vi "UTIL Generate Analog Output.vi"(6 "sampling info":cluster{"Fs":dbl, "#s":dbl}={"Fs"=1000.0, "#s"=1000.0} {"Fs" format="%.2p"}, 8 "error in (no error)":errorcluster, 9 "frequency":dbl=10.0 format="%0.2p", 10 "amplitude":dbl=1.0 format="%0.2p", 11 "task/channels in":refnum<k21>) -> (0 "error out":errorcluster, 3 "task out":refnum<k21>)   [LabVIEW 2010]
uses:
  <vilib>/DAQmx/write.llb/DAQmx Write (Analog Wfm 1Chan NSamp).vi
  <vilib>/daqmx/miscellaneous.llb/DAQmx Fill In Error Info.vi
  <vilib>/measure/NI_MABase.lvlib
panel:
  in  "stop":bool
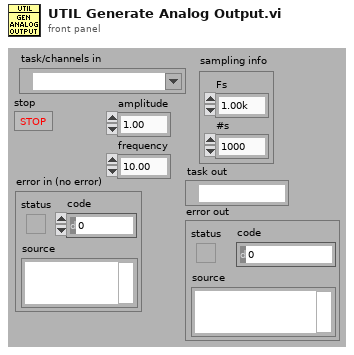
[diagram p1: front panel]
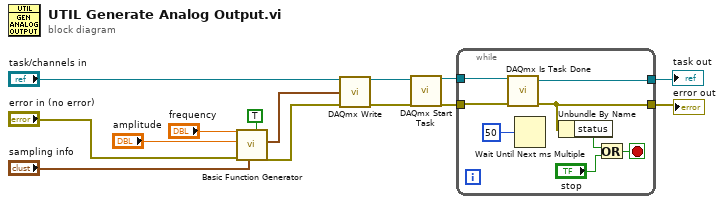
[diagram p0: block diagram]
diagram:
  n1 = call <vilib>:"Basic Function Generator.vi"("reset signal"=TRUE, "sampling info"="sampling info", "error in (no error)"="error in (no error)", "amplitude"="amplitude", "frequency"="frequency") -> ("error out"=w11:errorcluster, "signal out"=w10:waveform(dbl))  [unwired: 4 in, 1 out]
  n2 = call-poly <vilib>:"DAQmx Write.vi"("task/channels in"="task/channels in", "data"=w10, "error in"=w11) -> ("task out"=w8:refnum<k21>, "error out"=w9:errorcluster)  [unwired: 10 in, 1 out]
  n3 = call <vilib>:"DAQmx Start Task.vi"("task/channels in"=w8, "error in"=w9) -> ("task out"=w3:refnum<k21>, "error out"=w4:errorcluster)  [unwired: 12 in]
  n4 = while {
    tunnel: w3 -> [w22]
    tunnel: w4 -> [w21]
    tunnel: [w18] -> w2
    tunnel: [w19] -> w1
    stop <- w15 stop-if-true
    n5 = call <vilib>:"DAQmx Is Task Done.vi"("task/channels in"=w22, "error in"=w21) -> ("task out"=w19:refnum<k21>, "error out"=w18:errorcluster)  [unwired: 11 in, 1 out]
    n6 = Wait Until Next ms Multiple(millisecond multiple=u32 50) -> ()  [unwired: 1 out]
    n7 = Unbundle By Name(w18) -> ("status"=w16:bool)
    n8 = Or(x=w16, y="stop") -> (x .or. y?=w15:bool)
  }
  "task out" <- w1
  "error out" <- w2
